vi "format_arcmin2string.vi"() -> ()   [LabVIEW 2011]
panel:
  out "Arcmin":dbl format="%.2g"
  in  "Arcmin-Str":string
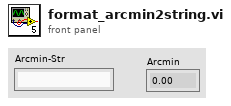
[diagram p1: front panel]
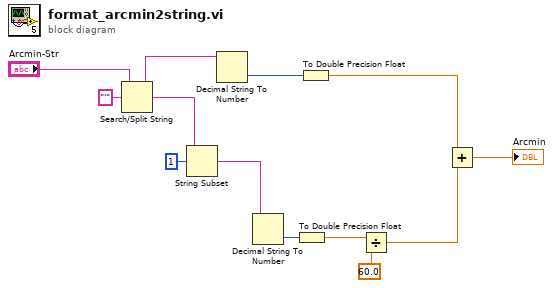
[diagram p0: block diagram]
diagram:
  n1 = Search/Split String(string="Arcmin-Str", search string/char (-)="'") -> (substring before match=w9:string, match + rest of string=w11:string)  [unwired: 1 in, 1 out]
  n2 = String Subset(string=w11, offset (0)=1) -> (substring=w8:string)  [unwired: 1 in]
  n3 = Decimal String To Number(string=w9) -> (number=w4:i32)  [unwired: 2 in, 1 out]
  n4 = Decimal String To Number(string=w8) -> (number=w7:i32)  [unwired: 2 in, 1 out]
  n5 = To Double Precision Float(number=w7) -> (double precision float=w6:dbl)
  n6 = To Double Precision Float(number=w4) -> (double precision float=w3:dbl)
  n7 = Divide(x=w6, y=60.0) -> (x/y=w2:dbl)
  n8 = Add(x=w3, y=w2) -> (x+y=→"Arcmin":dbl)
